vi "Gaussian_3(subVI).vi"(6 "Pulse Spacing (micro s)":dbl, 7 "Frequency (MHz)":dbl, 9 "Amplitude":dbl, 10 "Envelope Decay Time (micro s)":dbl, 11 "Number Of Points":i32) -> (3 "array":dbl[](array[numeric]))   [LabVIEW 2016]
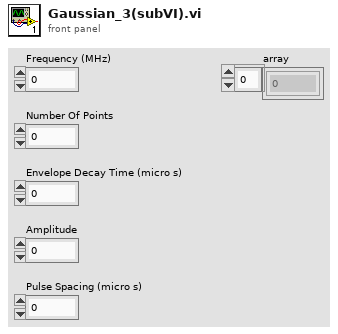
[diagram p1: front panel]
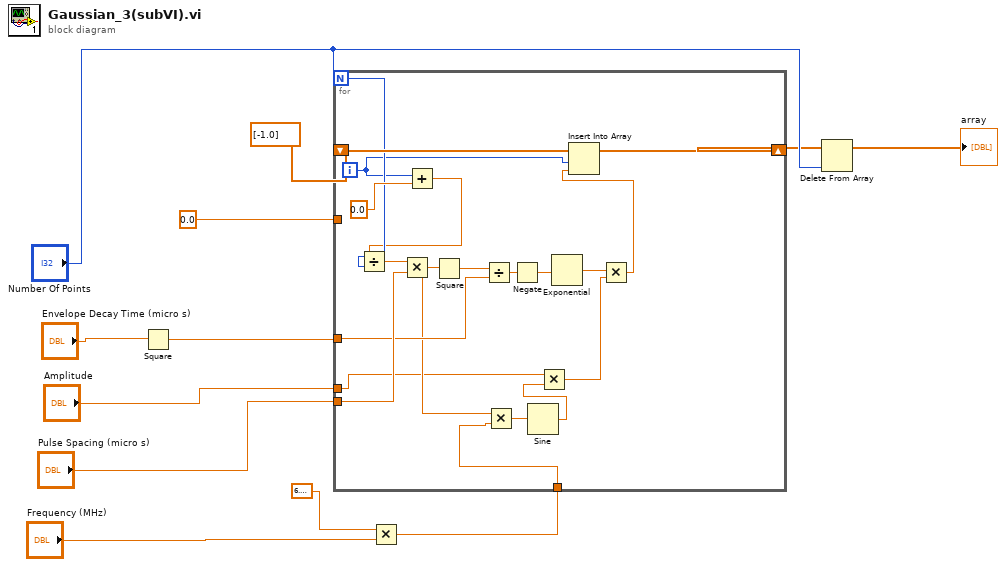
[diagram p0: block diagram]
diagram:
  n1 = Square(x="Envelope Decay Time (micro s)") -> (x^2=w5:dbl)
  n2 = Multiply(x=6.283185307179586, y="Frequency (MHz)") -> (x*y=w9:dbl)
  n3 = for {
    N: "Number Of Points" -> [w29]
    tunnel: "Amplitude" -> [w17]
    tunnel: "Pulse Spacing (micro s)" -> [w26]
    tunnel: 0.0 -> [_]
    shift-right: [w31] -> w6
    shift-left: dbl[] [-1.0] ("array") -> [w32]
    tunnel: w5 -> [w24]
    tunnel: w9 -> [w15]
    i -> [w19]
    n4 = Add(x=w19, y=0.0) -> (x+y=w28:dbl)
    n5 = Divide(x=w28, y=w29) -> (x/y=w27:dbl)
    n6 = Multiply(x=w27, y=w26) -> (x*y=w18:dbl)
    n7 = Square(x=w18) -> (x^2=w25:dbl)
    n8 = Divide(x=w25, y=w24) -> (x/y=w23:dbl)
    n9 = Multiply(x=w18, y=w15) -> (x*y=w14:dbl)
    n10 = Negate(x=w23) -> (-x=w22:dbl)
    n11 = Sine(x=w14) -> (sin(x)=w13:dbl)
    n12 = Multiply(x=w17, y=w13) -> (x*y=w16:dbl)
    n13 = Exponential(1:w22) -> (0:w21:dbl)
    n14 = Multiply(x=w21, y=w16) -> (x*y=w20:dbl)
    n15 = Insert Into Array(array=w32, index=w19, new element=w20) -> (w31:dbl[])
  }
  n16 = Delete From Array(array=w6, index="Number Of Points") -> (array with subset deleted=→"array":dbl[])  [unwired: 1 in, 1 out]
